vi "Read Bin.vi"(8 "Error In":errorcluster, 11 "Reader In":refnum<class "Reader.lvclass">) -> (0 "Error Out":errorcluster, 2 "Value":u8[](array[numeric]), 3 "Reader Out":refnum<class "Reader.lvclass">)   [LabVIEW 2019, in "LabPack.lvlib" / "Reader.lvclass"]
doc: "Reads and decodes a binary blob from the MessagePack data."
uses:
  Reader.lvclass
  Reader.lvclass/Reader.ctl
  Private/Read Bytes by Value.vi
  Private/Handle Error.vi
  Status/Read Status.vi
  Status/Read Status Message.vi
  Status/Read Is Error.vi
  Private/Begin Bin by Value.vi
  Utility/Status Code.vi
  <vilib>/Utility/error.llb/Error Cluster From Error Code.vi
  Private/End Bin by Value.vi
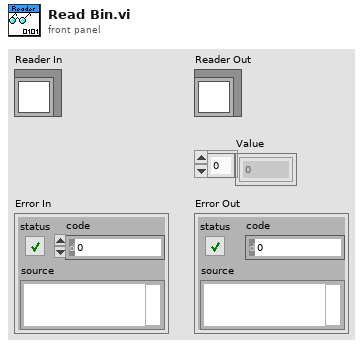
[diagram p1: front panel]
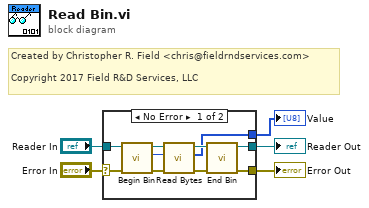
[diagram p0: block diagram]
diagram:
  # "Created by Christopher R. Field <chris@fieldrndservices.com>\n\nCopyright 2017 Field R&D Services, LLC"
  n1 = case shown="No Error" "Error In" {
    selector: "Error In" -> [w14 w16]
    tunnel: "Reader In" -> [w15 w17]
    tunnel: [w12 w16] -> w3
    tunnel: [w13 w17] -> w2
    tunnel: [w6 _] -> w1
    frame No Error {
      n2 = call-poly "Begin Bin.vi"("Error In"=w14, "Reader In"=w15) -> ("Error Out"=w10:errorcluster, "Count"=w9:u32, "Reader Out"=w11:refnum<class "Reader.lvclass">)  [unwired: 7 in]
      n3 = call-poly "Read Bytes.vi"("Error In"=w10, "Count"=w9, "Reader In"=w11) -> ("Error Out"=w7:errorcluster, "Bytes"=w6:u8[], "Reader Out"=w8:refnum<class "Reader.lvclass">)  [unwired: 6 in]
      n4 = call-poly "End Bin.vi"("Error In"=w7, "Reader In"=w8) -> ("Error Out"=w12:errorcluster, "Reader Out"=w13:refnum<class "Reader.lvclass">)  [unwired: 8 in]
    }
    frame Error {
    }
  }
  "Error Out" <- w3
  "Reader Out" <- w2
  "Value" <- w1
